vi "PID Calculate Outputs.vi"(9 "D Output":dbl, 10 "I Output":dbl, 11 "P Output":dbl) -> (3 "Output":dbl)   [LabVIEW 2014]
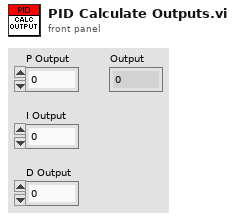
[diagram p1: front panel]
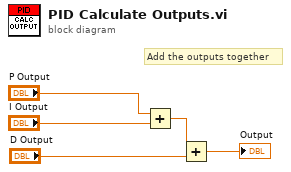
[diagram p0: block diagram]
diagram:
  # "Add the outputs together"
  n1 = Add(x="P Output", y="I Output") -> (x+y=w4:dbl)
  n2 = Add(x=w4, y="D Output") -> (x+y=→"Output":dbl)
